vi "DAQmxTask_Status.vi"(8 "error in (no error)":errorcluster caption="entrée d'erreur (pas d'erreur)", 11 "DAQmxTaskContainer_General en entrée":refnum<class "DAQmxTaksContainer_General.lvclass">) -> (0 "error out":errorcluster caption="sortie d'erreur", 1 "One at least active":bool, 2 "All active":bool, 3 "DAQmxTaskContainer_General en sortie":refnum<class "DAQmxTaksContainer_General.lvclass">)   [LabVIEW 2020, in "DAQmxTaksContainer_General.lvclass"]
uses:
  DAQmxTaksContainer_General.lvclass
  DAQmxTaksContainer_General.lvclass/DAQmxTaksContainer_General.ctl
  DAQmxTask.lvclass
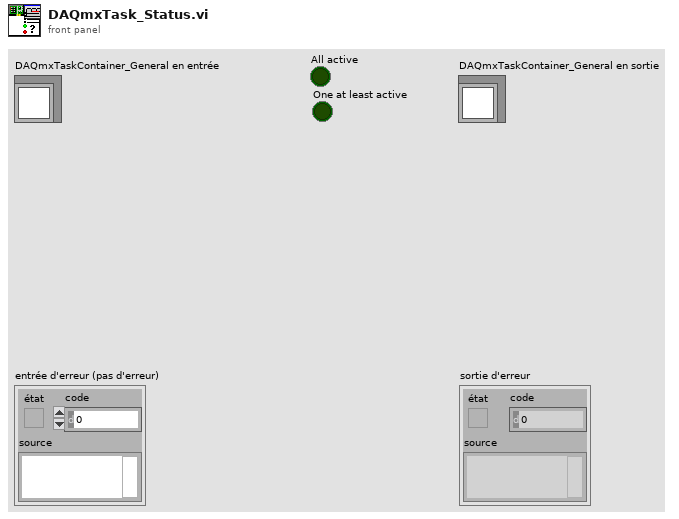
[diagram p1: front panel]
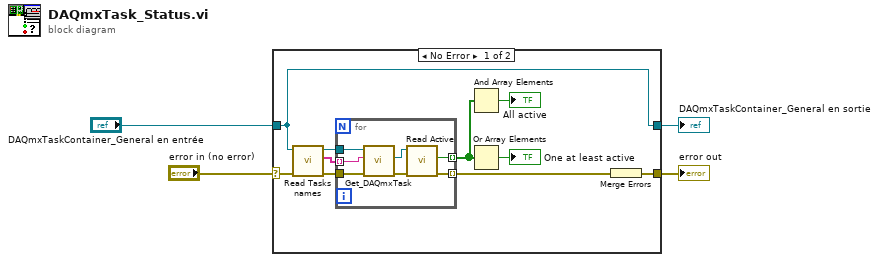
[diagram p0: block diagram]
diagram:
  n1 = case shown="No Error" "error in (no error)" {
    selector: "error in (no error)" -> [w14 w23]
    tunnel: [w9 w23] -> w3
    tunnel: [w12 w22] -> w1
    tunnel: "DAQmxTaskContainer_General en entrée" -> [w12 w22]
    frame No Error {
      n2 = call "Read Tasks names.vi"("error in (no error)"=w14, "DAQmxTaksContainer_General in"=w12) -> ("error out"=w10:errorcluster, "Tasks names"=w13:string[], "DAQmxTaksContainer_General out"=w11:refnum<class "DAQmxTaksContainer_General.lvclass">)  [unwired: 7 in]
      n3 = for {
        tunnel: w13 -> [w21] mode=indexing
        tunnel: w11 -> [w20]
        tunnel: w10 -> [w19]
        tunnel: [w16] -> w7 mode=indexing
        tunnel: [w15] -> w8 mode=indexing
        n4 = call "Get_DAQmxTask.vi"("error in (no error)"=w19, "Task name"=w21, "DAQmxTaksContainer_General in"=w20) -> ("error out"=w18:errorcluster, "DAQmx Task"=w17:refnum<class "DAQmxTask.lvclass">)  [unwired: 6 in, 1 out]
        n5 = call-dynamic "Read Active.vi"("error in (no error)"=w18, "DAQmxTask in"=w17) -> ("error out"=w15:errorcluster, "Active?"=w16:bool)  [unwired: 7 in, 1 out]
      }
      n6 = And Array Elements(Boolean array=w7) -> (logical AND=→"All active":bool)
      n7 = Or Array Elements(Boolean array=w7) -> (logical OR=→"One at least active":bool)
      n8 = Merge Errors(w8) -> (w9:errorcluster)
    }
    frame Error {
    }
  }
  "error out" <- w3
  "DAQmxTaskContainer_General en sortie" <- w1
